vi "SavePhoto.vi"(11 "Instrument path":path) -> (3 "Instrument out":path)   [LabVIEW 2022 SP3]
panel:
  in  "Add":bool
  out "Image":picture
  in  "Image path":path
  # "Select a path (click on the folder icon to the right or just drag a file on to the Image path control)"
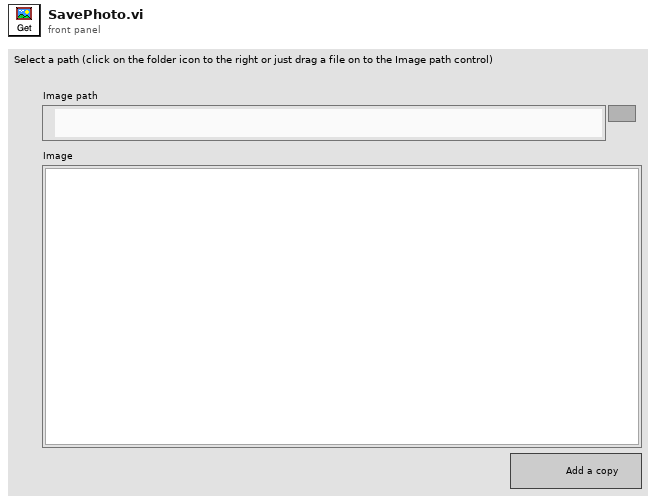
[diagram p1: front panel]
types:
  T1 = typedef "LVBoundsTypeDef.ctl" = cluster{"Width":u32, "Height":u32}
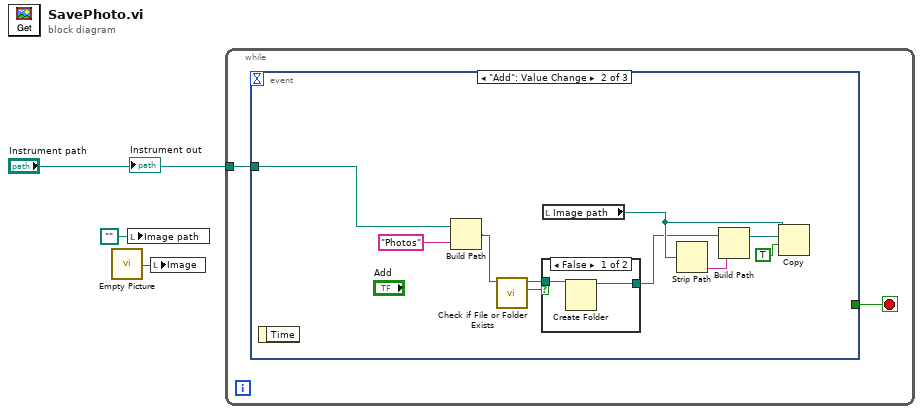
[diagram p0: block diagram]
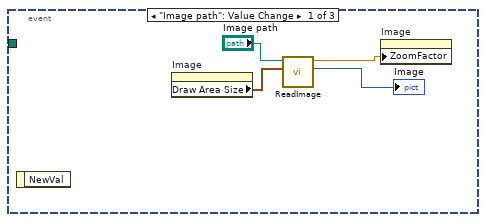
[diagram p2: hidden frame]
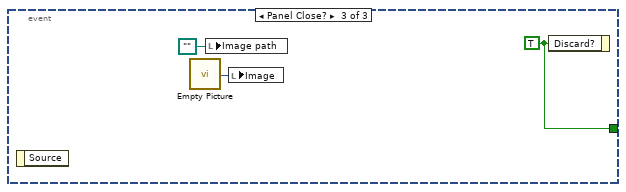
[diagram p4: hidden frame]
diagram:
  n1 = call "Empty Picture"() -> ("empty picture"=w3:picture)
  n2 = local write "Image path"(path "" ("Image path")) -> ()
  n3 = local write "Image"(w3) -> ()
  n4 = while {
    tunnel: "Instrument path" -> [w4]
    stop <- w5 stop-if-true
    n5 = event shown="[1] \"Add\": Value Change" {
      selector: _ -> [_ _ _]
      dyn-events: _ -> [_ _ _]
      timeout: _ -> [_ _ _]
      tunnel: [_ _ w25] -> w5
      tunnel: w4 -> [_ w10 _]
      event "Image path": Value Change {
        n6 = event-data() -> ()  [unwired: 1 in, 1 out]
        n7 = property on="Image" class="Pict"() -> ("Draw Area Size"=w8:T1)  [unwired: 2 in, 2 out]
        n8 = call "ReadImage.vi"("Draw Area Size"=w8, "Image path"="Image path") -> ("Image"=→"Image":picture, "zoom"=w7:dbl)  [unwired: 7 in, 1 out]
        n9 = property on="Image" class="Pict"("ZoomFactor"=w7) -> ()  [unwired: 2 in, 2 out]
      }
      event "Add": Value Change {
        n10 = event-data() -> ()  [unwired: 1 in, 1 out]
        n11 = Build Path(base path=w10, name or relative path="Photos") -> (appended path=w13:path)
        n12 = call <vilib>:"Check if File or Folder Exists.vi"("path"=w13) -> ("file or folder exists?"=w14:bool, "dup path"=w12:path)  [unwired: 8 in, 1 out]
        n13 = case shown="False" w14 {
          tunnel: w12 -> [w21 w22]
          tunnel: [w20 w22] -> w11
          frame False {
            n14 = Create Folder(path (use dialog)=w21) -> (created path=w20:path)  [unwired: 2 in, 2 out]
          }
          frame True {
          }
        }
        n15 = local read "Image path"() -> (w18:path)
        n16 = Strip Path(path=w18) -> (name=w17:string)  [unwired: 1 out]
        n17 = Build Path(base path=w11, name or relative path=w17) -> (appended path=w16:path)
        n18 = Copy(9:TRUE ("overwrite (F)"), 10:w16, 11:w18) -> ()  [unwired: 2 in, 3 out]
      }
      event Panel Close? {
        w25 = TRUE ("Discard?")
        n19 = event-data() -> ()  [unwired: 1 in, 1 out]
        n20 = call "Empty Picture"() -> ("empty picture"=w23:picture)
        n21 = local write "Image path"(path "" ("Image path")) -> ()
        n22 = local write "Image"(w23) -> ()
        n23 = event-data("Discard?"=w25) -> ()  [unwired: 1 in, 1 out]
      }
    }
  }
  "Instrument out" <- "Instrument path"
